vi "Send Text Message.vi"(8 "error in":errorcluster, 10 "body":string, 11 "subject":string) -> (0 "error out":errorcluster)   [LabVIEW 2017]
uses:
  <vilib>/smtpClient/Set Message Text.vi
  <vilib>/smtpClient/LabVIEWSMTPClient.lvlib
panel:
  in  "Email info":T1={"server address"="smtp.gmail.com:587", "email"="jiaruiyang123@gmail.com", "password"="HYsheng1024"}
  in  "phone SMTP gateway":string="2403705359@messaging.sprintpcs.com"
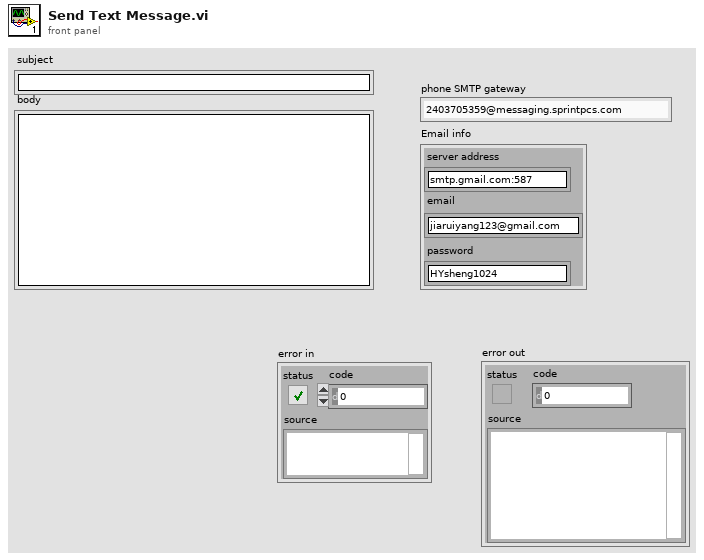
[diagram p1: front panel]
types:
  T1 = cluster{"server address":string, "email":string, "password":string}
  T2 = typedef "LabVIEWSMTPClient.lvlib/SmtpClientHandle.ctl" = refnum<k1>
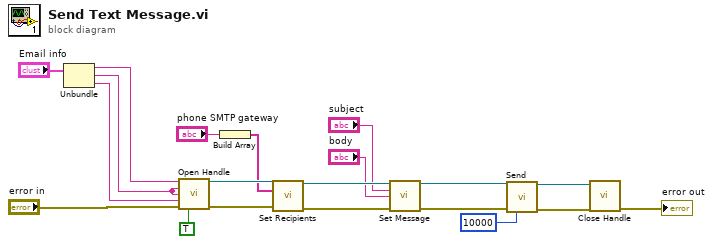
[diagram p0: block diagram]
diagram:
  n1 = Unbundle("Email info") -> ("server address"=w3:string, "email"=w2:string, "password"=w1:string)
  n2 = call <vilib>:"Open Handle.vi"("server address"=w3, "from"=w2, "username"=w2, "password"=w1, "error in (no error)"="error in", "use TLS (false)"=TRUE) -> ("handle out"=w8:T2, "error out"=w19:errorcluster)  [unwired: 8 in]
  n3 = Build Array("phone SMTP gateway") -> (w7:string[])
  n4 = call <vilib>:"Set Recipients.vi"("handle in"=w8, "to"=w7, "error in (no error)"=w19) -> ("handle out"=w11:T2, "error out"=w18:errorcluster)  [unwired: 11 in]
  n5 = call-poly <vilib>:"Set Message.vi"("handle in"=w11, "subject"="subject", "plain text message"="body", "error in (no error)"=w18) -> ("handle out"=w12:T2, "error out"=w17:errorcluster)  [unwired: 10 in]
  n6 = call <vilib>:"Send.vi"("handle in"=w12, "error in (no error)"=w17, "timeout in ms (10000)"=10000) -> ("handle out"=w13:T2, "error out"=w16:errorcluster)  [unwired: 10 in, 1 out]
  n7 = call <vilib>:"Close Handle.vi"("handle in"=w13, "error in (no error)"=w16) -> ("error out"=→"error out":errorcluster)  [unwired: 12 in, 1 out]
